vi "MDS_Main.vi"() -> ()   [LabVIEW 2025]
uses:
  Builds/Queue Wrappers.lvlibp
  Libraries/Queue Wrappers/Q Wrappers.lvlib
panel:
  in  "Tab":enum32{"Page 1", "Page 2", "Status Log"}(tab)
  out "Status Log":cluster{"Status Log":string, "Path":path}
  in  "Transfer Settings":bool
  in  "Stop User Events":bool
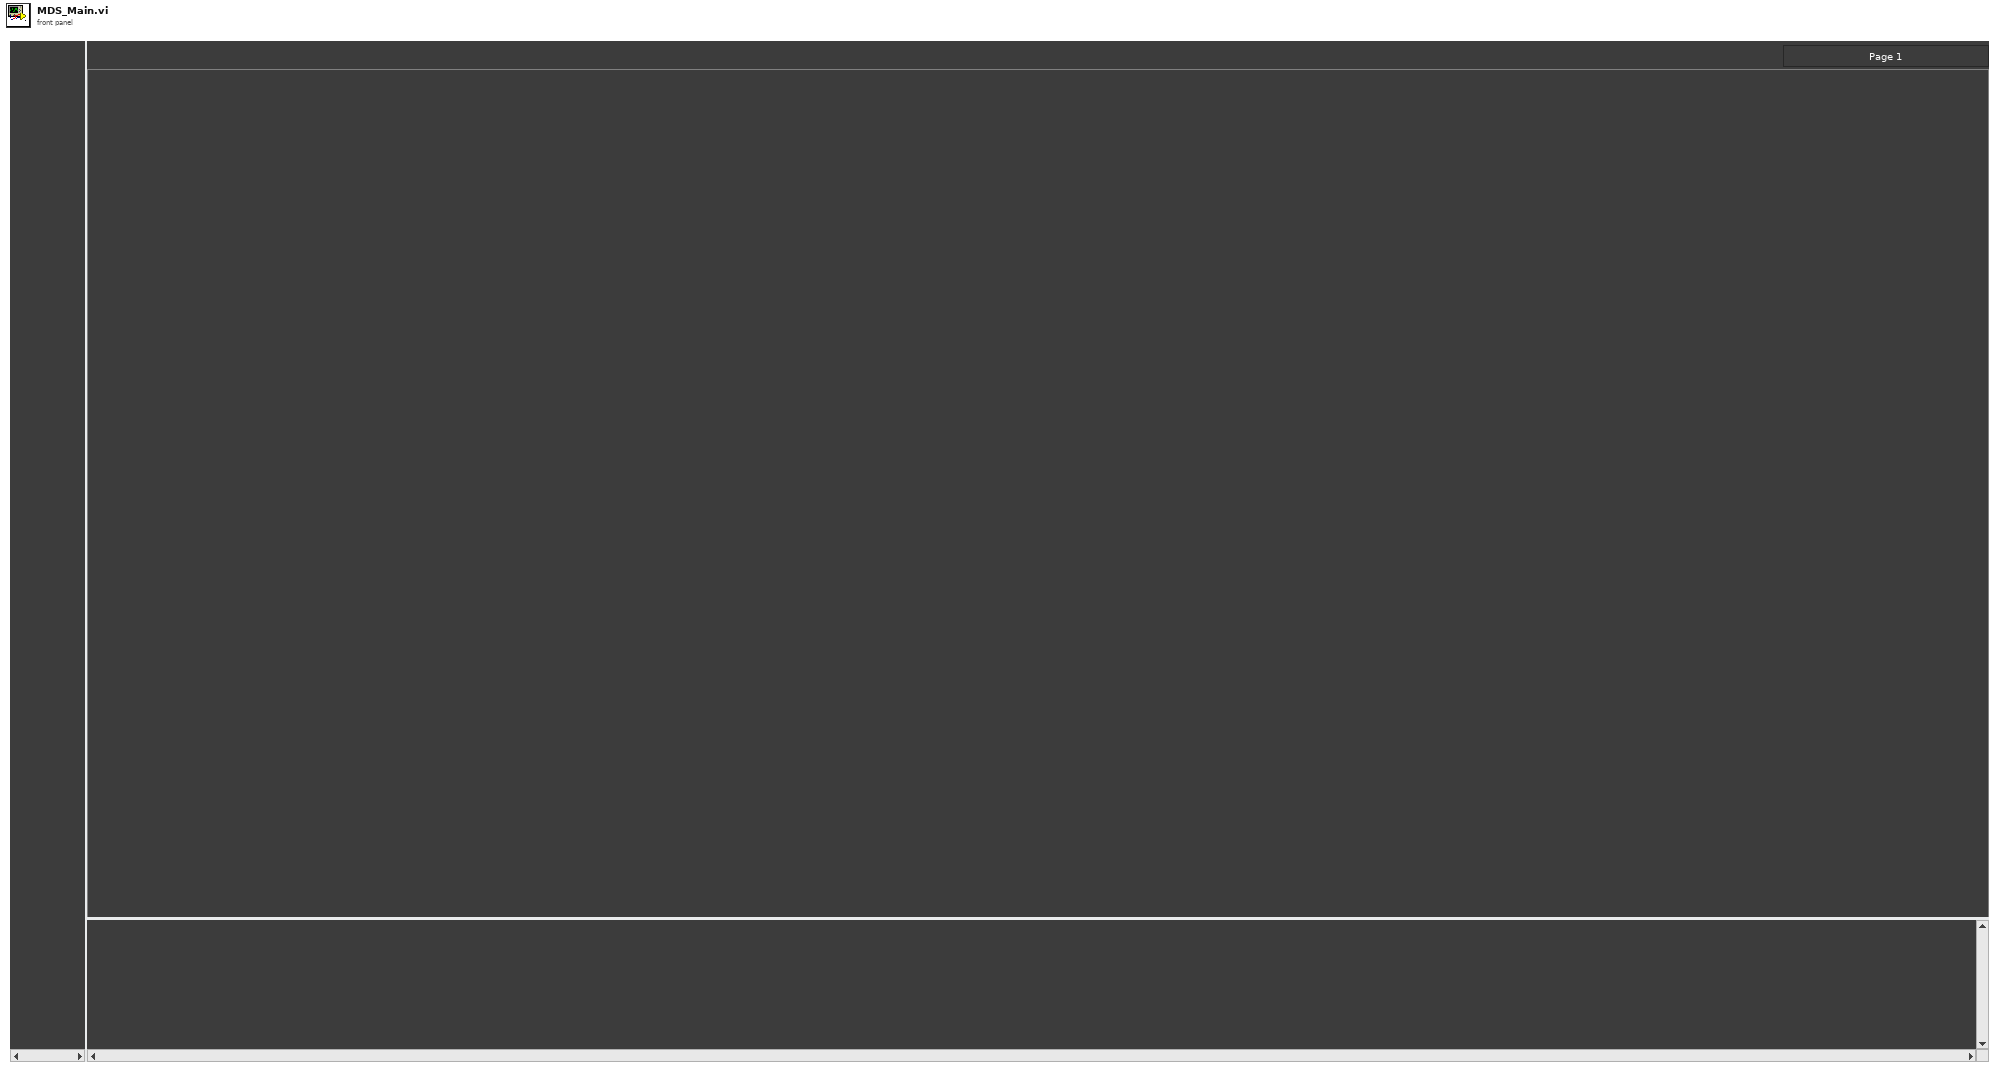
[diagram p1: front panel]
types:
  T1 = typedef "Queues-Refs-Data.ctl" = cluster{"Queues":cluster{"Operations":refnum<queue>, "Acquisition":refnum<queue>, "Processing":refnum<queue>, "Recording":refnum<queue>, "Display":refnum<queue>, "Data Out":refnum<queue>, "Messages In":refnum<queue>, "Messages Out":refnum<queue>, "Errors":refnum<queue>}, "Refs":cluster{"Main VI":refnum<vi>, "Stop User Events":refnum<vi>, "Transfer Settings":refnum<vi>, "Status Log":refnum<vi>, "Tab":refnum<vi>}, "Data":cluster{"Software ID":string, "Software Version":string, "Status Log Directory":path, "Status Log File":path}}
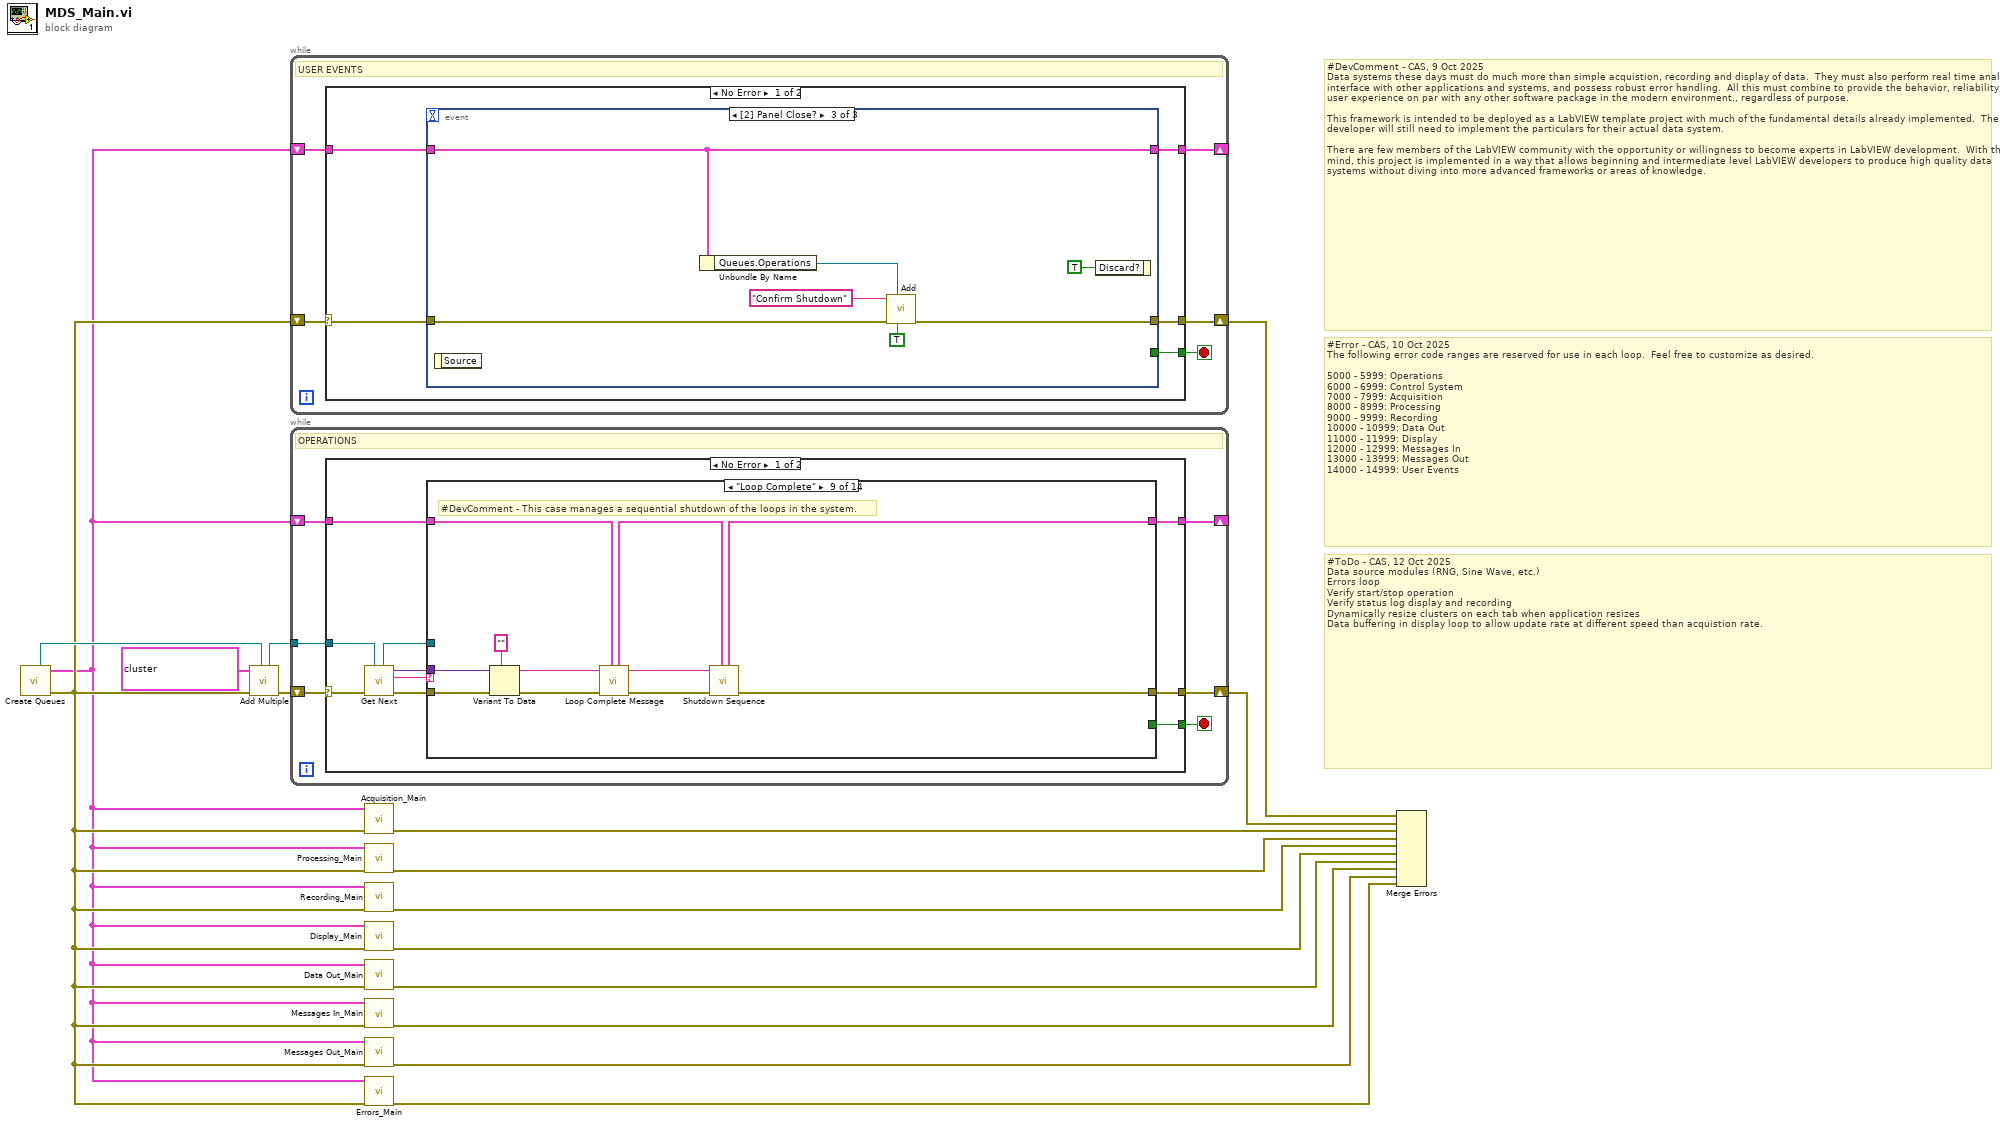
[diagram p0: block diagram]
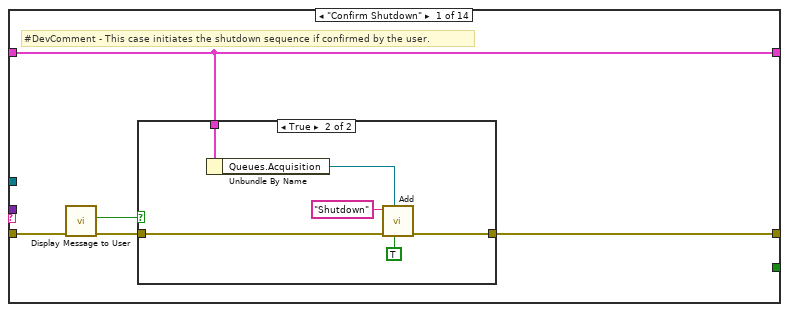
[diagram p2: hidden frame]
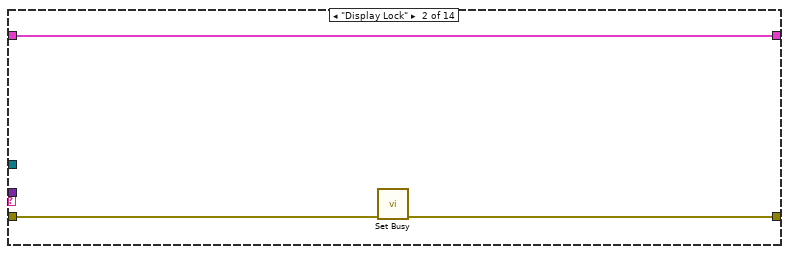
[diagram p4: hidden frame]
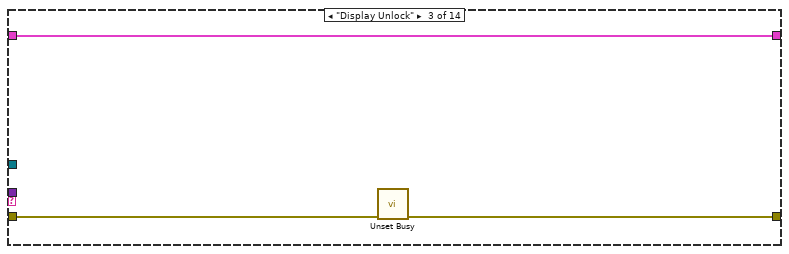
[diagram p5: hidden frame]
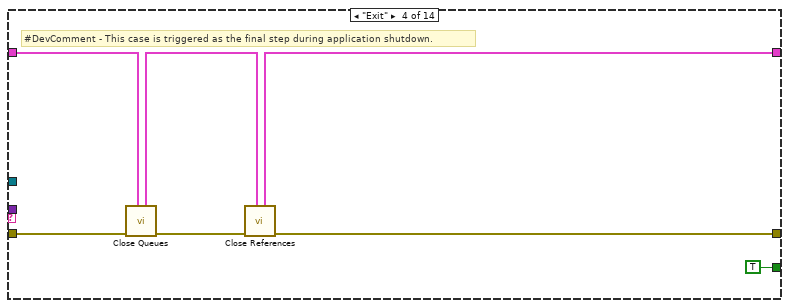
[diagram p6: hidden frame]
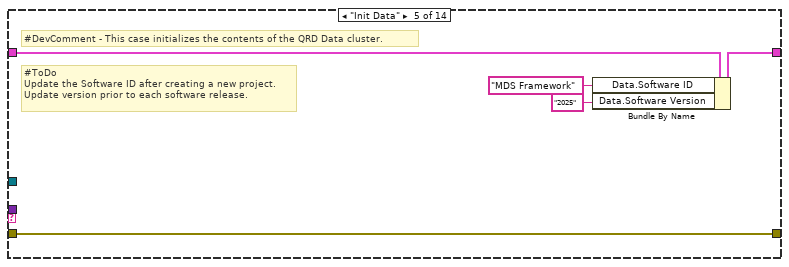
[diagram p7: hidden frame]
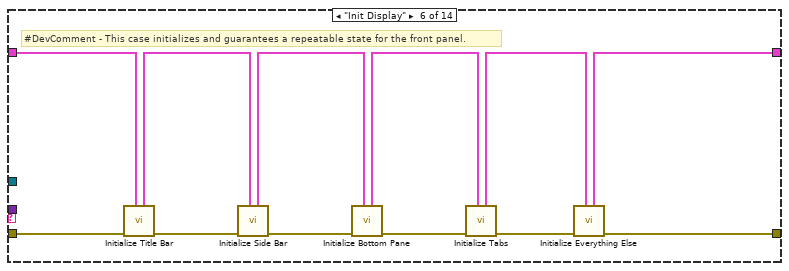
[diagram p8: hidden frame]
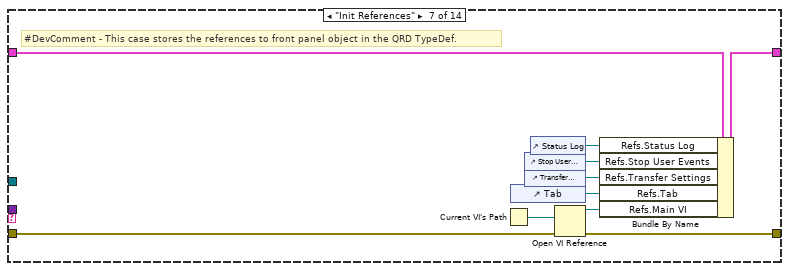
[diagram p9: hidden frame]
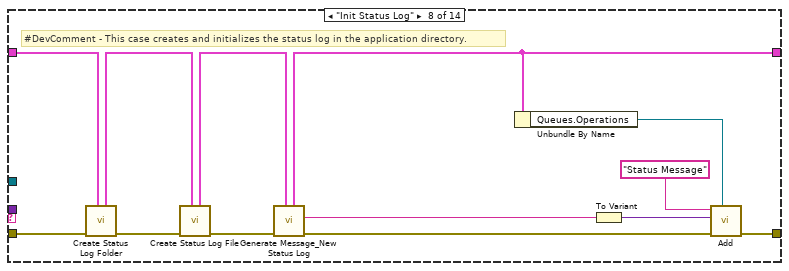
[diagram p10: hidden frame]
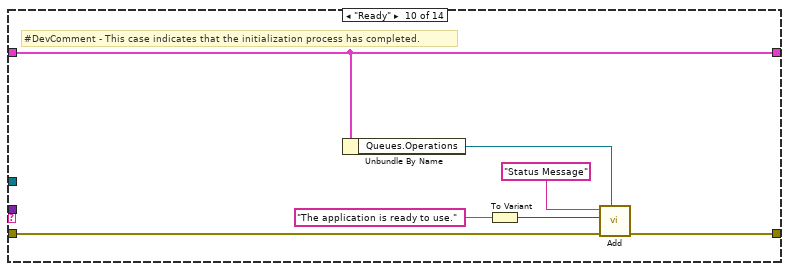
[diagram p11: hidden frame]
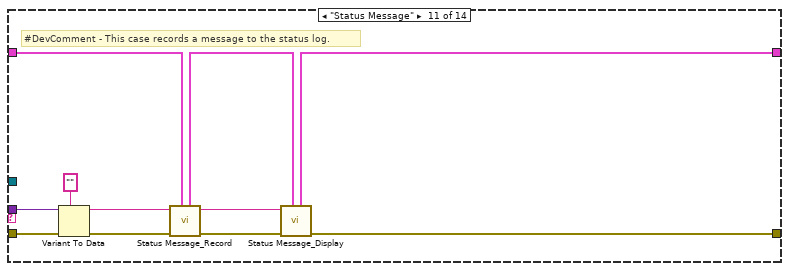
[diagram p12: hidden frame]
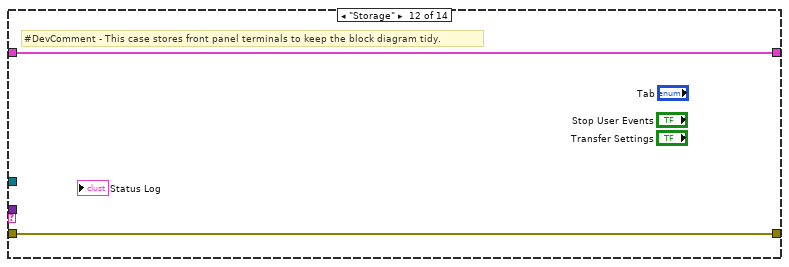
[diagram p13: hidden frame]
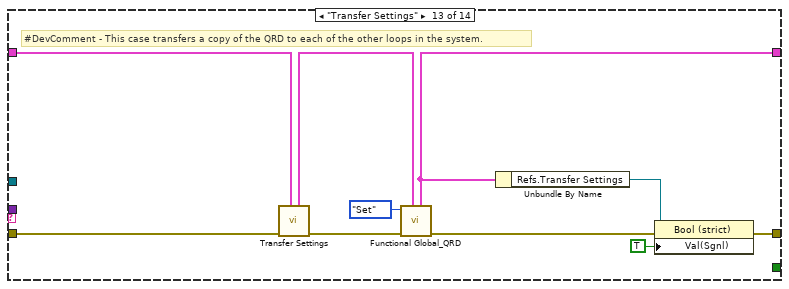
[diagram p14: hidden frame]
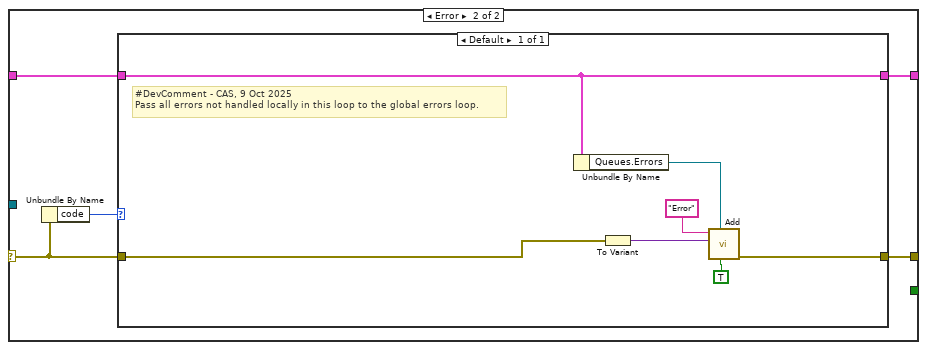
[diagram p16: hidden frame]
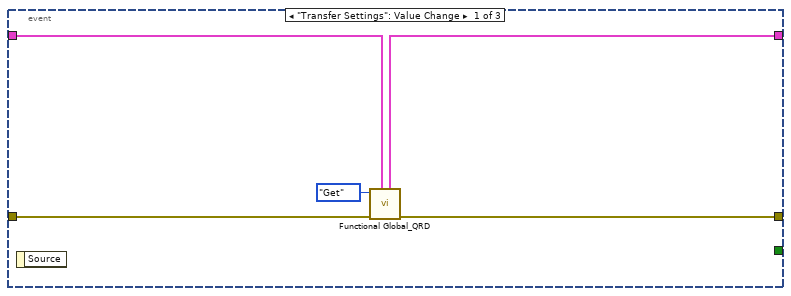
[diagram p17: hidden frame]
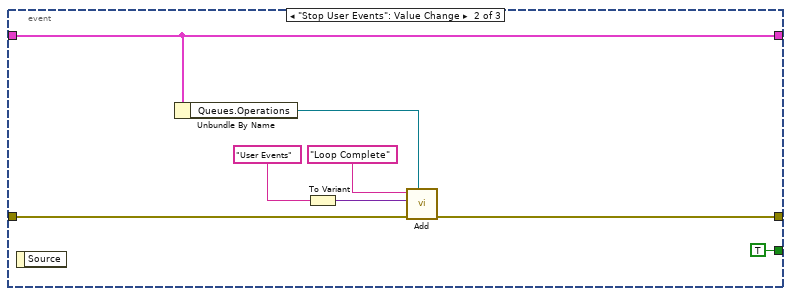
[diagram p18: hidden frame]
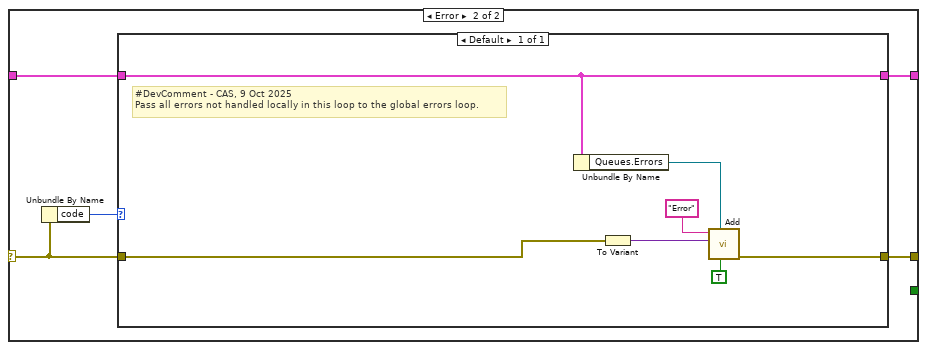
[diagram p19: hidden frame]
diagram:
  # "#ToDo - CAS, 12 Oct 2025\nData source modules (RNG, Sine Wave, etc.)\nErrors loop\nVerify start/stop operation\nVerify status log display and recording\nDynamically resize clusters on each tab when application resizes\nData buffering in display loop to allow update rate at different speed than acquistion rate."
  # "#Error - CAS, 10 Oct 2025\nThe following error code ranges are reserved for use in each loop.  Feel free to customize as desired.\n\n5000 - 5999: Operations\n6000 - 6999: Control System\n7000 - 7999: Acquisition\n8000 - 8999: Processing\n9000 - 9999: Recording\n10000 - 10999: Data Out\n11000 - 11999: Display\n12000 - 12999: Messages In\n13000 - 13999: Messages Out\n14000 - 14999: User Events"
  # "#DevComment - CAS, 9 Oct 2025\nData systems these days must do much more than simple acquistion, recording and display of data.  They must also perform real time analysis, interface with other applications and systems, and possess robust error handling.  All this must combine to provide the behavior, reliability, and user experience on par with any other software package in the modern environment., regardless of purpose.\n\nThis framework is intended to be deployed as a LabVIEW template project with much of the fundamental details already implemented.  The end developer will still need to implement the particulars for their actual data system.\n\nThere are few members of the LabVIEW community with the opportunity or willingness to become experts in LabVIEW development.  With that in mind, this project is implemented in a way that allows beginning and intermediate level LabVIEW developers to produce high quality data systems without diving into more advanced frameworks or areas of knowledge."
  n1 = call "Create Queues.vi"() -> ("error out"=w2:errorcluster, "QRD Out"=w1:T1, "Operations Q"=w16:refnum<queue>)  [unwired: 9 in]
  n2 = call "Add Multiple.vi"("Q Ref In"=w16, "error in"=w2, "Q Packets"=cluster{"Packet ID":string, "Payload":variant}[] [{"Packet ID"="Display Lock", "Payload"=variant}, {"Packet ID"="Init References", "Payload"=variant}, {"Packet ID"="Init Data", "Payload"=variant}, {"Packet ID"="Init Status Log", "Payload"=variant}, {"Packet ID"="Init Display", "Payload"=variant}, {"Packet ID"="Display Unlock", "Payload"=variant}, {"Packet ID"="Transfer Settings", "Payload"=variant}, {"Packet ID"="Ready", "Payload"=variant}]) -> ("error out"=w14:errorcluster, "Q Ref Out"=w15:refnum<queue>)  [unwired: 7 in]
  n3 = while {
    shift-right: [w19] -> w13
    shift-left: w2 -> [w20]
    shift-right: [w18] -> _
    shift-left: w1 -> [w21]
    stop <- w17 stop-if-true
    # "USER EVENTS"
    n4 = case shown="No Error" w20 {
      selector: w20 -> [w26 w50]
      tunnel: w21 -> [w25 w48]
      tunnel: [w24 w47] -> w19
      tunnel: [w23 w49] -> w18
      tunnel: [w22 _] -> w17
      frame No Error {
        n5 = event shown="[2] Panel Close?" {
          selector: _ -> [_ _ _]
          dyn-events: _ -> [_ _ _]
          timeout: _ -> [_ _ _]
          tunnel: w26 -> [w29 w38 w44]
          tunnel: w25 -> [w27 w37 w42]
          tunnel: [w30 w39 w43] -> w24
          tunnel: [w28 w37 w42] -> w23
          tunnel: [_ TRUE ("Discard?") _] -> w22
          event "Transfer Settings": Value Change {
            n6 = event-data() -> ()  [unwired: 1 in, 1 out]
            n7 = call "Functional Global_QRD.vi"("QRD"=w27, "error in"=w29, "Function"=enum16{"Set", "Get"}."Get") -> ("error out"=w30:errorcluster, "QRD Out"=w28:T1)  [unwired: 7 in]
          }
          event "Stop User Events": Value Change {
            n8 = event-data() -> ()  [unwired: 1 in, 1 out]
            n9 = Unbundle By Name(w37) -> ("Queues.Operations"=w36:refnum<queue>)
            n10 = To Variant(anything="User Events" ("Packet ID")) -> (Variant=w34:variant)
            n11 = call "Add.vi"("Q Ref In"=w36, "error in"=w38, "Payload"=w34, "Packet ID"="Loop Complete") -> ("error out"=w39:errorcluster)  [unwired: 4 in, 3 out]
          }
          event Panel Close? {
            n12 = event-data() -> ()  [unwired: 1 in, 1 out]
            n13 = Unbundle By Name(w42) -> ("Queues.Operations"=w41:refnum<queue>)
            n14 = call "Add.vi"("Priority Message"=TRUE, "Q Ref In"=w41, "error in"=w44, "Packet ID"="Confirm Shutdown") -> ("error out"=w43:errorcluster)  [unwired: 4 in, 3 out]
            n15 = event-data("Discard?"=TRUE) -> ()  [unwired: 1 in, 1 out]
          }
        }
      }
      frame Error {
        n16 = Unbundle By Name(w50) -> ("code"=w51:i32)
        n17 = case shown="Default" w51 {
          tunnel: w50 -> [w57]
          tunnel: [w58] -> w49
          tunnel: w48 -> [w58]
          tunnel: [w55] -> w47
          frame Default {
            # "#DevComment - CAS, 9 Oct 2025\nPass all errors not handled locally in this loop to the global errors loop."
            n18 = Unbundle By Name(w58) -> ("Queues.Errors"=w52:refnum<queue>)
            n19 = To Variant(anything=w57) -> (Variant=w54:variant)
            n20 = call "Add.vi"("Priority Message"=TRUE, "Q Ref In"=w52, "Payload"=w54, "Packet ID"="Error") -> ("error out"=w55:errorcluster)  [unwired: 4 in, 3 out]
          }
        }
      }
    }
  }
  n21 = while {
    shift-right: [w62] -> w12
    shift-left: w14 -> [w63]
    shift-right: [w61] -> _
    shift-left: w1 -> [w64]
    tunnel: w15 -> [w60]
    stop <- w59 stop-if-true
    # "OPERATIONS"
    n22 = case shown="No Error" w63 {
      selector: w63 -> [w71 w186]
      tunnel: w64 -> [w74 w184]
      tunnel: [w72 w183] -> w62
      tunnel: [w73 w185] -> w61
      tunnel: w60 -> [w67 _]
      tunnel: [w66 _] -> w59
      frame No Error {
        n23 = call "Get Next.vi"("Q Ref In"=w67, "error in"=w71) -> ("error out"=w70:errorcluster, "Packet ID"=w69:string, "Payload"=w65:variant, "Q Ref Out"=w68:refnum<queue>)  [unwired: 6 in]
        n24 = case shown="\"Loop Complete\"" w69 {
          tunnel: w68 -> [_ _ _ _ _ _ _ _ _ _ _ _ _ _]
          tunnel: w70 -> [w79 w88 w91 w96 w104 w116 w126 w139 w150 w156 w168 w169 w174 w181]
          tunnel: w74 -> [w76 w89 w92 w93 w102 w115 w122 w138 w140 w154 w158 w170 w171 w182]
          tunnel: [w76 w89 w92 w98 w103 w105 w123 w127 w145 w154 w164 w170 w179 w182] -> w73
          tunnel: [w75 w87 w90 w97 w104 w107 w125 w133 w147 w155 w167 w169 w176 w181] -> w72
          tunnel: [_ _ _ TRUE _ _ _ _ _ _ _ _ _ _] -> w66
          tunnel: w65 -> [_ _ _ _ _ _ _ _ w149 _ w165 _ _ _]
          frame "Confirm Shutdown" {
            # "#DevComment - This case initiates the shutdown sequence if confirmed by the user."
            n25 = call "Display Message to User"("error in (no error)"=w79) -> ("error out"=w78:errorcluster, "OK"=w77:bool)  [unwired: 9 in]
            n26 = case shown="True" w77 {
              tunnel: w78 -> [w80 w86]
              tunnel: w76 -> [_ w85]
              tunnel: [w80 w83] -> w75
              frame False {
              }
              frame True {
                n27 = Unbundle By Name(w85) -> ("Queues.Acquisition"=w84:refnum<queue>)
                n28 = call "Add.vi"("Priority Message"=TRUE, "Q Ref In"=w84, "error in"=w86, "Packet ID"="Shutdown") -> ("error out"=w83:errorcluster)  [unwired: 4 in, 3 out]
              }
            }
          }
          frame "Display Lock" {
            n29 = call <vilib>:"Set Busy.vi"("error in (no error)"=w88) -> ("error out"=w87:errorcluster)  [unwired: 9 in, 1 out]
          }
          frame "Display Unlock" {
            n30 = call <vilib>:"Unset Busy.vi"("error in (no error)"=w91) -> ("error out"=w90:errorcluster)  [unwired: 10 in]
          }
          frame "Exit" {
            # "#DevComment - This case is triggered as the final step during application shutdown."
            n31 = call "Close Queues.vi"("QRD"=w93, "error in"=w96) -> ("error out"=w95:errorcluster, "QRD Out"=w94:T1)  [unwired: 8 in]
            n32 = call "Close References.vi"("QRD"=w94, "error in"=w95) -> ("error out"=w97:errorcluster, "QRD Out"=w98:T1)  [unwired: 8 in]
          }
          frame "Init Data" {
            # "#DevComment - This case initializes the contents of the QRD Data cluster."
            # "#ToDo\nUpdate the Software ID after creating a new project.\nUpdate version prior to each software release."
            n33 = Bundle By Name(cluster=w102, "Data.Software ID"="MDS Framework", "Data.Software Version"="2025") -> (w103:T1)
          }
          frame "Init Display" {
            # "#DevComment - This case initializes and guarantees a repeatable state for the front panel."
            n34 = call "Initialize Title Bar.vi"("QRD"=w115, "error in"=w116) -> ("error out"=w114:errorcluster, "QRD Out"=w113:T1)  [unwired: 8 in]
            n35 = call "Initialize Side Bar.vi"("QRD"=w113, "error in"=w114) -> ("error out"=w112:errorcluster, "QRD Out"=w110:T1)  [unwired: 8 in]
            n36 = call "Initialize Bottom Pane.vi"("QRD"=w110, "error in"=w112) -> ("error out"=w111:errorcluster, "QRD Out"=w109:T1)  [unwired: 8 in]
            n37 = call "Initialize Tabs.vi"("QRD"=w109, "error in"=w111) -> ("error out"=w108:errorcluster, "QRD Out"=w106:T1)  [unwired: 8 in]
            n38 = call "Initialize Everything Else.vi"("QRD"=w106, "error in"=w108) -> ("error out"=w107:errorcluster, "QRD Out"=w105:T1)  [unwired: 8 in]
          }
          frame "Init References" {
            # "#DevComment - This case stores the references to front panel object in the QRD TypeDef."
            n39 = Current VI's Path() -> (path=w124:path)
            n40 = control-ref of="Tab"() -> (w120:refnum<vi>)
            n41 = control-ref of="Stop User Events"() -> (w118:refnum<vi>)
            n42 = control-ref of="Transfer Settings"() -> (w119:refnum<vi>)
            n43 = control-ref of="Status Log"() -> (w117:refnum<vi>)
            n44 = Open VI Reference(vi path=w124, error in (no error)=w126) -> (vi reference=w121:refnum<vi>, error out=w125:errorcluster)  [unwired: 4 in]
            n45 = Bundle By Name(cluster=w122, "Refs.Status Log"=w117, "Refs.Stop User Events"=w118, "Refs.Transfer Settings"=w119, "Refs.Tab"=w120, "Refs.Main VI"=w121) -> (w123:T1)
          }
          frame "Init Status Log" {
            # "#DevComment - This case creates and initializes the status log in the application directory."
            n46 = call "Create Status Log Folder.vi"("QRD"=w138, "error in"=w139) -> ("error out"=w137:errorcluster, "QRD Out"=w136:T1)  [unwired: 8 in]
            n47 = call "Create Status Log File.vi"("QRD"=w136, "error in"=w137) -> ("error out"=w131:errorcluster, "QRD Out"=w130:T1)  [unwired: 8 in]
            n48 = call "Generate Message_New Status Log.vi"("QRD"=w130, "error in"=w131) -> ("error out"=w128:errorcluster, "Status Log Message"=w129:string, "QRD Out"=w127:T1)  [unwired: 7 in]
            n49 = Unbundle By Name(w127) -> ("Queues.Operations"=w135:refnum<queue>)
            n50 = To Variant(anything=w129) -> (Variant=w132:variant)
            n51 = call "Add.vi"("Q Ref In"=w135, "error in"=w128, "Payload"=w132, "Packet ID"="Status Message") -> ("error out"=w133:errorcluster)  [unwired: 4 in, 3 out]
          }
          frame "Loop Complete" {
            # "#DevComment - This case manages a sequential shutdown of the loops in the system."
            n52 = Variant To Data(error in=w150, type="", Variant=w149) -> (data=w143:string, error out=w148:errorcluster)
            n53 = call "Loop Complete Message.vi"("QRD"=w140, "error in"=w148, "Loop ID"=w143) -> ("error out"=w144:errorcluster, "Loop ID Out"=w142:string, "QRD Out"=w141:T1)  [unwired: 6 in]
            n54 = call "Shutdown Sequence.vi"("QRD"=w141, "error in"=w144, "Loop ID"=w142) -> ("error out"=w147:errorcluster, "QRD Out"=w145:T1)  [unwired: 7 in]
          }
          frame "Ready" {
            # "#DevComment - This case indicates that the initialization process has completed."
            n55 = Unbundle By Name(w154) -> ("Queues.Operations"=w153:refnum<queue>)
            n56 = To Variant(anything="The application is ready to use." ("Packet ID")) -> (Variant=w151:variant)
            n57 = call "Add.vi"("Q Ref In"=w153, "error in"=w156, "Payload"=w151, "Packet ID"="Status Message") -> ("error out"=w155:errorcluster)  [unwired: 4 in, 3 out]
          }
          frame "Status Message" {
            # "#DevComment - This case records a message to the status log."
            n58 = Variant To Data(error in=w168, type="", Variant=w165) -> (data=w161:string, error out=w163:errorcluster)
            n59 = call "Status Message_Record.vi"("QRD"=w158, "error in"=w163, "Status Message"=w161) -> ("error out"=w162:errorcluster, "Status Message Out"=w160:string, "QRD Out"=w159:T1)  [unwired: 6 in]
            n60 = call "Status Message_Display.vi"("QRD"=w159, "error in"=w162, "Status Message"=w160) -> ("error out"=w167:errorcluster, "QRD Out"=w164:T1)  [unwired: 7 in]
          }
          frame "Storage" {
            # "#DevComment - This case stores front panel terminals to keep the block diagram tidy."
          }
          frame "Transfer Settings" {
            # "#DevComment - This case transfers a copy of the QRD to each of the other loops in the system."
            n61 = call "Transfer Settings.vi"("QRD"=w171, "error in"=w174) -> ("error out"=w173:errorcluster, "QRD Out"=w172:T1)  [unwired: 8 in]
            n62 = call "Functional Global_QRD.vi"("QRD"=w172, "error in"=w173, "Function"=enum16{"Set", "Get"}."Set") -> ("error out"=w177:errorcluster, "QRD Out"=w179:T1)  [unwired: 7 in]
            n63 = Unbundle By Name(w179) -> ("Refs.Transfer Settings"=w178:refnum<vi>)
            n64 = property class="Bool (strict)"(reference=w178, error in=w177, "Val(Sgnl)"=TRUE ("Value (Signaling)")) -> (error out=w176:errorcluster)  [unwired: 1 out]
          }
          frame Default {
          }
        }
      }
      frame Error {
        n65 = Unbundle By Name(w186) -> ("code"=w187:i32)
        n66 = case shown="Default" w187 {
          tunnel: w186 -> [w193]
          tunnel: [w194] -> w185
          tunnel: w184 -> [w194]
          tunnel: [w190] -> w183
          frame Default {
            # "#DevComment - CAS, 9 Oct 2025\nPass all errors not handled locally in this loop to the global errors loop."
            n67 = Unbundle By Name(w194) -> ("Queues.Errors"=w189:refnum<queue>)
            n68 = To Variant(anything=w193) -> (Variant=w191:variant)
            n69 = call "Add.vi"("Priority Message"=TRUE, "Q Ref In"=w189, "Payload"=w191, "Packet ID"="Error") -> ("error out"=w190:errorcluster)  [unwired: 4 in, 3 out]
          }
        }
      }
    }
  }
  n70 = call "Acquisition_Main.vi"("error in"=w2, "QRD"=w1) -> ("error out"=w11:errorcluster)  [unwired: 9 in]
  n71 = call "Processing_Main.vi"("error in"=w2, "QRD"=w1) -> ("error out"=w3:errorcluster)  [unwired: 9 in]
  n72 = call "Recording_Main.vi"("error in"=w2, "QRD"=w1) -> ("error out"=w10:errorcluster)  [unwired: 9 in]
  n73 = call "Display_Main.vi"("error in"=w2, "QRD"=w1) -> ("error out"=w9:errorcluster)  [unwired: 9 in]
  n74 = call "Data Out_Main.vi"("error in"=w2, "QRD"=w1) -> ("error out"=w8:errorcluster)  [unwired: 9 in]
  n75 = call "Messages In_Main.vi"("error in"=w2, "QRD"=w1) -> ("error out"=w6:errorcluster)  [unwired: 9 in]
  n76 = call "Messages Out_Main.vi"("error in"=w2, "QRD"=w1) -> ("error out"=w7:errorcluster)  [unwired: 9 in]
  n77 = call "Errors_Main.vi"("error in"=w2, "QRD"=w1) -> ("error out"=w5:errorcluster)  [unwired: 9 in]
  n78 = Merge Errors(w13, w12, w11, w3, w10, w9, w8, w6, w7, w5) -> ()  [unwired: 1 out]
